vi "ReadChangedLibrariesLog.vi"(8 "error in (no error)":errorcluster) -> (0 "error out":errorcluster, 3 "ChangedLibraries":string[](array[string]))   [LabVIEW 2023, in "CICD.lvlib"]
uses:
  CICD.lvlib
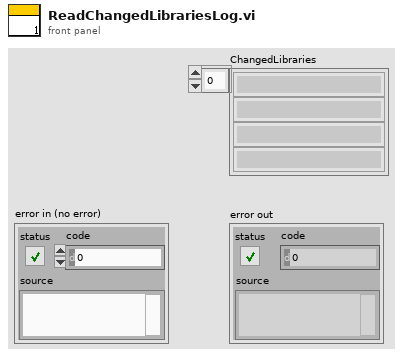
[diagram p1: front panel]
types:
  T1 = enum16{"open", "replace", "create", "open or create", "replace or create", "replace or create with confirmation"}
  T2 = typedef "CICD.lvlib/CICDPathConfigs.ctl" = cluster{"GlobalIncludePaths":path[], "GlobalExcludePaths":path[], "BuildSpecsIncludePaths":path[], "ActualDepsIncludePaths":path[], "WorkspacePath":path, "SourceFolderPaths":path[], "ChangedFilesLogpaths":map{string, path}}
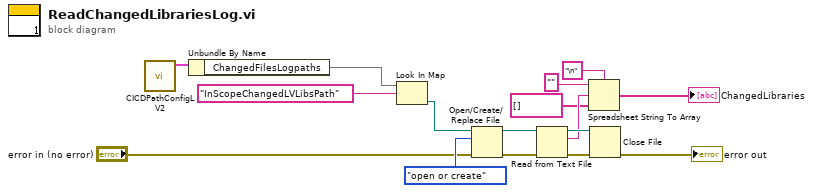
[diagram p0: block diagram]
diagram:
  n1 = call "CICDPathConfigLV2.vi"() -> ("CICD Path Config Out"=w16:T2)  [unwired: 11 in]
  n2 = Unbundle By Name(w16) -> ("ChangedFilesLogpaths"=w14:map{string, path})
  n3 = Look In Map(map=w14, key="InScopeChangedLVLibsPath") -> (value=w6:path)  [unwired: 1 in, 1 out]
  n4 = Open/Create/Replace File(file path (use dialog)=w6, error in="error in (no error)", operation (0:open)=T1."open or create") -> (refnum out=w12:refnum<file>, error out=w11:errorcluster)  [unwired: 3 in, 1 out]
  n5 = Read from Text File(file (use dialog)=w12, error in=w11) -> (refnum out=w10:refnum<file>, text=w8:string, error out=w9:errorcluster)  [unwired: 2 in, 1 out]
  n6 = Spreadsheet String To Array(delimiter (Tab)="\n", format string="", spreadsheet string=w8, array type (2D Dbl)=string[] []) -> (array=→"ChangedLibraries":string[])
  n7 = Close File(refnum=w10, error in=w9) -> (error out=→"error out":errorcluster)  [unwired: 1 out]
